vi "Write My Data to CSV (empty).vi"(4 "Data":T1(array[cluster]), 5 "Comment":string, 7 "Time Stamp":timestamp, 8 "error in":errorcluster, 11 "file path":path) -> (0 "error out":errorcluster)   [LabVIEW 2011]
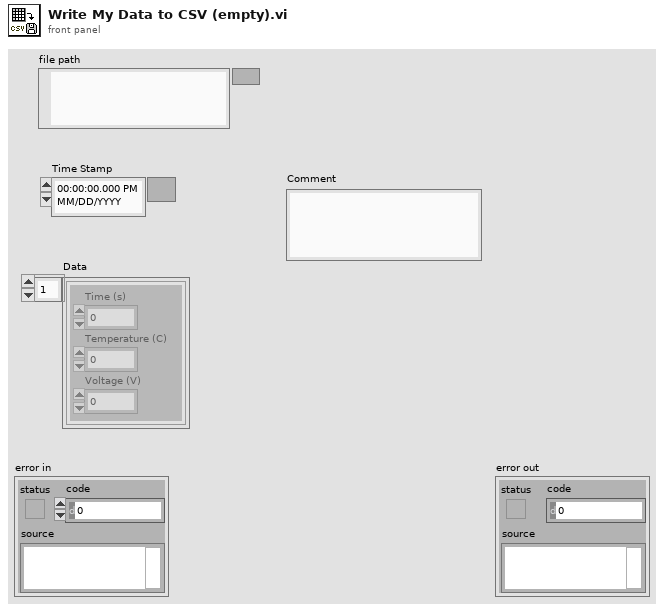
[diagram p1: front panel]
types:
  T1 = cluster{"Time (s)":dbl, "Temperature (C)":dbl, "Voltage (V)":dbl}[]
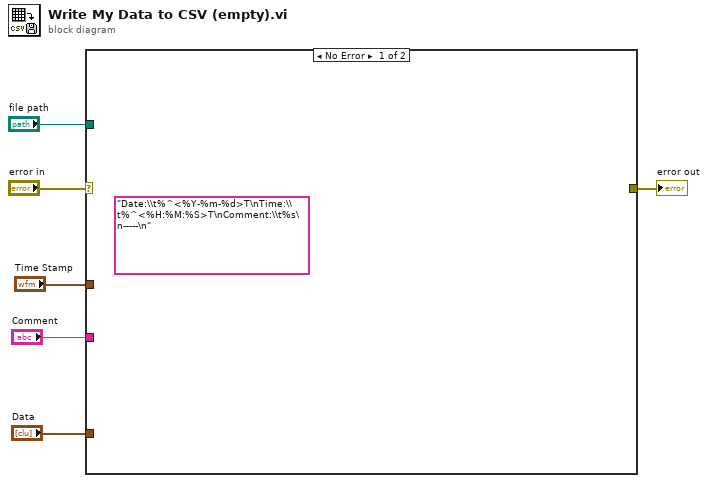
[diagram p0: block diagram]
diagram:
  n1 = case shown="No Error" "error in" {
    selector: "error in" -> [_ w7]
    tunnel: "Data" -> [_ _]
    tunnel: [_ w7] -> w6
    tunnel: "file path" -> [_ _]
    tunnel: "Time Stamp" -> [_ _]
    tunnel: "Comment" -> [_ _]
    frame No Error {
      (unwired) "Date:\\t%^<%Y-%m-%d>T\nTime:\\t%^<%H:%M:%S>T\nComment:\\t%s\n-----\n" ("format string")
    }
    frame Error {
      # "Wire previous error through"
    }
  }
  "error out" <- w6
